vi "GetHelp.vi"(11 "RunVI in":refnum<class "RunVI.lvclass">) -> (2 "Help":string, 3 "RunVI out":refnum<class "RunVI.lvclass">)   [LabVIEW 2014, in "RunVI.lvclass"]
uses:
  RunVI.lvclass
panel:
  in  "Help":string="LabVIEWCLI -OperationName RunVI -VIPath <path of the vi to run> <arguments>\n -VIPath\t\tPath of the VI to run. For the connector pane of this VI, please refer how to use document.\n <arguments>\t\tArray of string which will be passed to the VI."
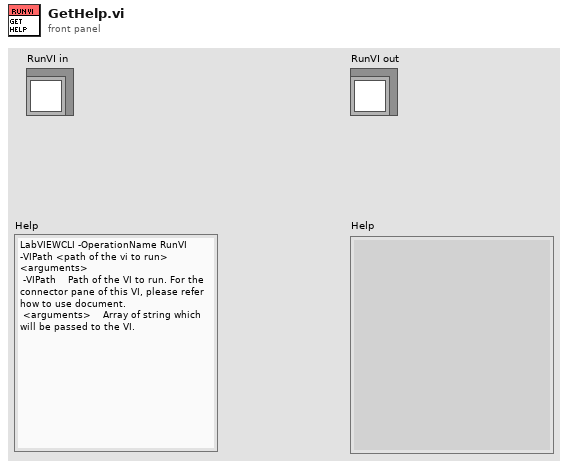
[diagram p1: front panel]
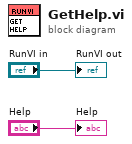
[diagram p0: block diagram]
diagram:
  "RunVI out" <- "RunVI in"
  "Help" <- "Help"
